vi "measure frequency response.vi"(0 "AWG Visa Name":refnum<visa-resource-name>="AWG5014", 1 "Amp 1":dbl=1.0, 2 "Amp 2":dbl=1.0, 3 "Wipe Names on execute":bool, 5 "Cant. Freq":dbl=5000.0, 7 "Frequency":dbl=40000000.0, 11 "LIA VISA Name":refnum<visa-resource-name>, 12 "Single Lock-in Parameter 2 (0: X output)":i32(ring)=3 items=["X output", "Y output", "R output", "Theta output", "Aux In 1", "Aux In 2", "Aux In 3", "Aux In 4", "Aux Out 1", "Aux Out 2", "Xnoise", "Ynoise", "Reference Phase", "Sine Out Amplitude", "DC Level", "Int. Ref. Frequency", "Ext. Ref. Frequency"], 13 "Single Lock-in Parameter (0: X output)":u16(ring)=2 items=["X output", "Y output", "R output", "Theta output", "Aux In 1", "Aux In 2", "Aux In 3", "Aux In 4", "Aux Out 1", "Aux Out 2", "Xnoise", "Ynoise", "Reference Phase", "Sine Out Amplitude", "DC Level", "Int. Ref. Frequency", "Ext. Ref. Frequency"]) -> (8 "Output Value(2 parameters)":cluster{"Value 1":dbl, "Value 2":dbl}, 15 "error out":errorcluster)   [LabVIEW 2018]
uses:
  <instrlib>/Stanford Research SR865/Stanford Research SR865.lvlib
panel:
  in  "Reference Source (0: Internal)":i32(ring)=1 items=["Internal", "External", "Dual", "Chop"]
  in  "Ref. Name":string="lorem"
  in  "Sum Name":string="ipsum"
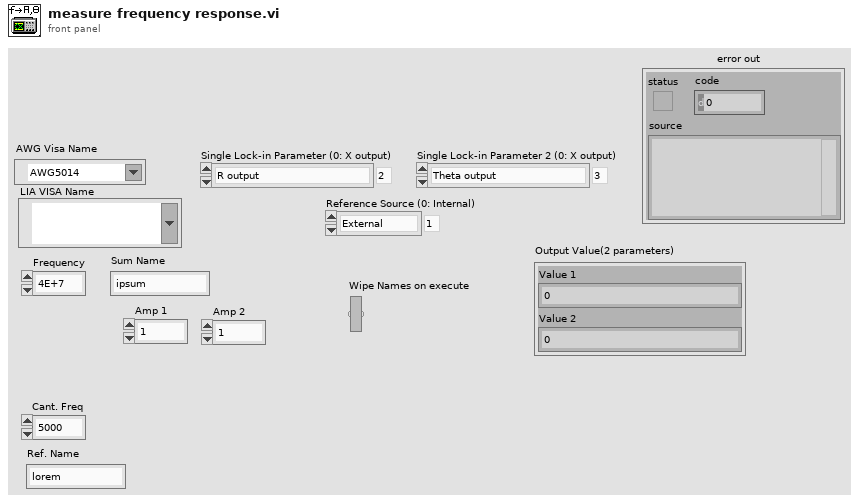
[diagram p1: front panel]
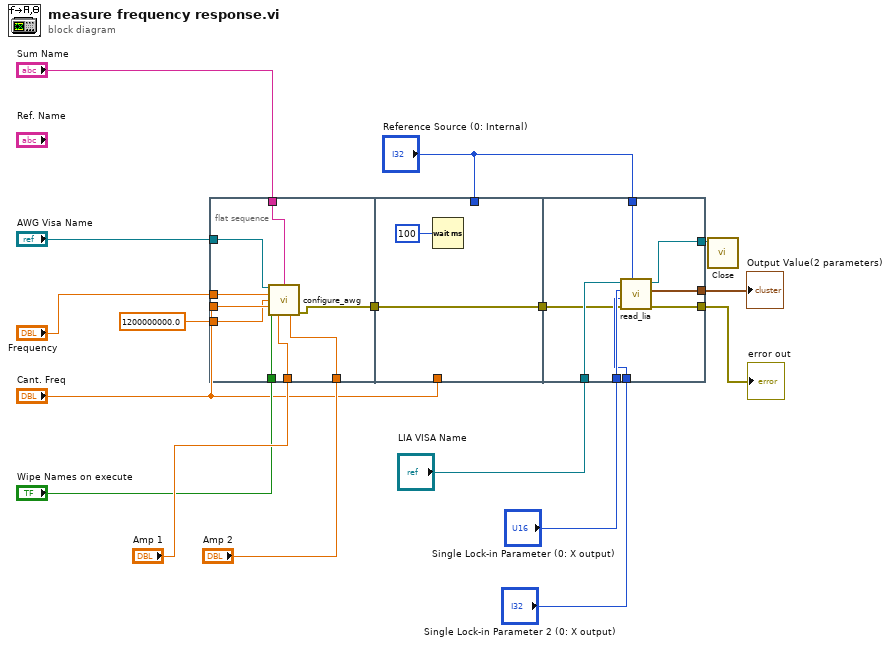
[diagram p0: block diagram]
diagram:
  n1 = flat-sequence {
    tunnel: "Amp 2" -> [w26]
    tunnel: "Amp 1" -> [w25]
    tunnel: "Wipe Names on execute" -> [w24]
    tunnel: "Cant. Freq" -> [w23]
    tunnel: "Sum Name" -> [w22]
    tunnel: "Frequency" -> [w21]
    tunnel: "AWG Visa Name" -> [w20]
    tunnel: 1200000000.0 ("Max sample rate") -> [w19]
    tunnel: [w18] -> w2
    tunnel: "Reference Source (0: Internal)" -> [_]
    tunnel: "Cant. Freq" -> [_]
    tunnel: [w27] -> w3
    tunnel: w2 -> [w27]
    tunnel: "Reference Source (0: Internal)" -> [w36]
    tunnel: "Single Lock-in Parameter (0: X output)" -> [w35]
    tunnel: "Single Lock-in Parameter 2 (0: X output)" -> [w34]
    tunnel: [w33] -> w10
    tunnel: [w32] -> w9
    tunnel: "LIA VISA Name" -> [w31]
    tunnel: w3 -> [w30]
    tunnel: [w29] -> w1
    frame #0 {
      n2 = call "configure_awg.vi"("VISA name"=w20, "Sum Name"=w22, "Frequency"=w21, "Max sample rate"=w19, "Cant. Freq"=w23, "Wipe Names on execute"=w24, "Amp 1"=w25, "Amp 2"=w26) -> ("error out"=w18:errorcluster)  [unwired: 7 in]
    }
    frame #1 {
      n3 = Wait (ms)(milliseconds to wait=u32 100) -> ()  [unwired: 1 out]
    }
    frame #2 {
      n4 = call "read_lia.vi"("Reference Source (0: Internal)"=w36, "error in (no error)"=w30, "Single Lock-in Parameter 2 (0: X output)"=w34, "Single Lock-in Parameter (0: X output)"=w35, "VISA resource name"=w31) -> ("error out"=w29:errorcluster, "Output Value(2 parameters)"=w33:cluster{"Value 1":dbl, "Value 2":dbl}, "VISA resource name out"=w32:refnum<visa-resource-name>)  [unwired: 4 in]
    }
  }
  n5 = call <instrlib>:"Close.vi"("VISA resource name"=w9) -> ()  [unwired: 10 in, 1 out]
  "Output Value(2 parameters)" <- w10
  "error out" <- w1
